vi "Day 12 Clusters and Enums.vi"() -> ()   [LabVIEW 2026]
uses:
  State_Machine_States.ctl
panel:
  in  "Measurement Record Database":T1(array[cluster])
  in  "Enum 2":T2=enum."Idle"
  out "Action Command":string
  in  "Enum":enum16{"RED", "YELLOW", "GREEN"}(ring)
  in  "First name 3":string
  out "Age 2":dbl
  out "First name 2":string
  out "Female":bool
  out "Age":dbl
  out "Last name":string
  out "First name":string
  in  "Cluster":T3
  # "Cluster for a measurement record"
  # "EXPLOARATION OF CLUSTER DATA TYPE"
  # "type-def enum"
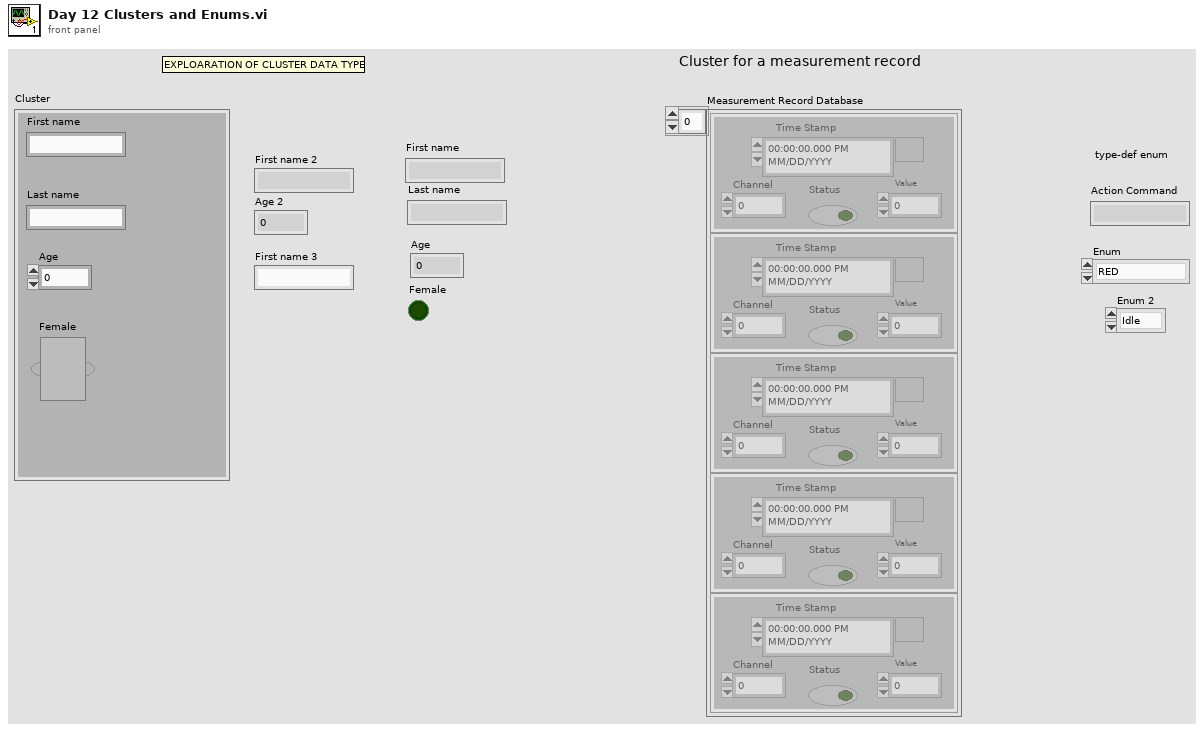
[diagram p1: front panel]
types:
  T1 = cluster{"Time Stamp":timestamp, "Channel":dbl, "Value":dbl, "Status":bool}[]
  T2 = typedef "State_Machine_States.ctl" = enum16{"TRIAL", "Idle", "Configuring", "Processing", "Error"}
  T3 = cluster{"First name":string, "Last name":string, "Age":dbl, "Female":bool}
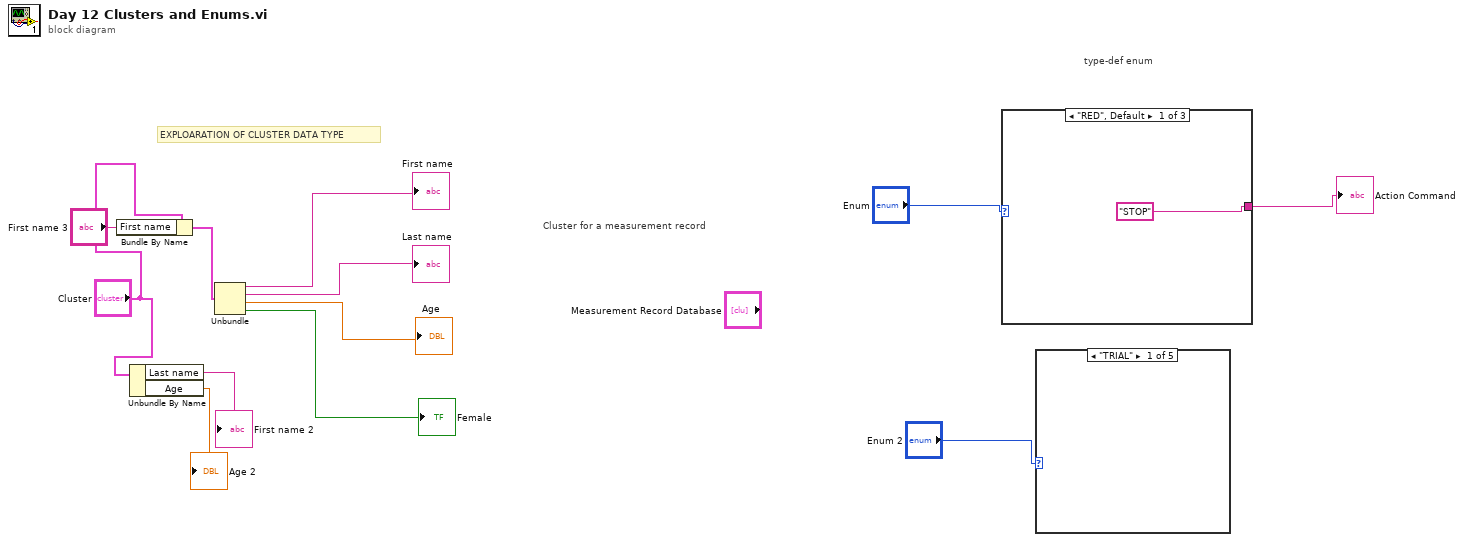
[diagram p0: block diagram]
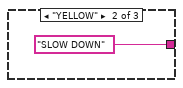
[diagram p6: hidden frame]
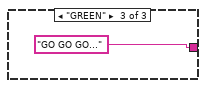
[diagram p7: hidden frame]
diagram:
  # "type-def enum"
  # "Cluster for a measurement record"
  # "EXPLOARATION OF CLUSTER DATA TYPE"
  n1 = Bundle By Name "Bundle By Name"(cluster="Cluster", "First name"="First name 3") -> (w4:T3)
  n2 = Unbundle By Name "Unbundle By Name"("Cluster") -> ("Last name"=→"First name 2":string, "Age"=→"Age 2":dbl)
  n3 = Unbundle "Unbundle"(w4) -> ("First name"=→"First name":string, "Last name"=→"Last name":string, "Age"=→"Age":dbl, "Female"=→"Female":bool)
  n4 = case shown="\"RED\", Default" "Enum" {
    tunnel: ["STOP" "SLOW DOWN" "GO GO GO..."] -> w2
    frame "RED", Default {
    }
    frame "YELLOW" {
    }
    frame "GREEN" {
    }
  }
  "Action Command" <- w2
  n5 = case shown="\"TRIAL\"" "Enum 2" {
    frame "TRIAL" {
    }
    frame "Idle", Default {
    }
    frame "Configuring" {
    }
    frame "Processing" {
    }
    frame "Error" {
    }
  }
